vi "DriveSpeed.vi"(8 "R In":dbl, 9 "Y In":dbl, 10 "X In":dbl, 11 "Half Speed":bool) -> (1 "R Out":dbl, 2 "Y Out":dbl, 3 "X Out":dbl)   [LabVIEW 2014]
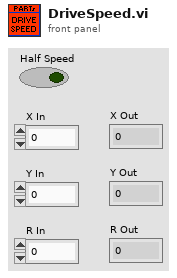
[diagram p1: front panel]
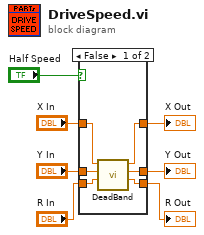
[diagram p0: block diagram]
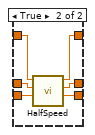
[diagram p2: hidden frame]
diagram:
  n1 = case shown="False" "Half Speed" {
    tunnel: "X In" -> [w13 w19]
    tunnel: "Y In" -> [w12 w18]
    tunnel: "R In" -> [w11 w17]
    tunnel: [w10 w16] -> w3
    tunnel: [w9 w15] -> w2
    tunnel: [w8 w14] -> w1
    frame False {
      n2 = call "DeadBand.vi"("R In"=w11, "Y In"=w12, "X In"=w13) -> ("R Out"=w8:dbl, "Y Out"=w9:dbl, "X Out"=w10:dbl)  [unwired: 6 in]
    }
    frame True {
      n3 = call "HalfSpeed.vi"("R In"=w17, "Y In"=w18, "X In"=w19) -> ("R Out"=w14:dbl, "Y Out"=w15:dbl, "X Out"=w16:dbl)  [unwired: 6 in]
    }
  }
  "X Out" <- w3
  "Y Out" <- w2
  "R Out" <- w1
